vi "VCS Stop Recorder.vi"(8 "error in (no error)":errorcluster, 11 "axis in":cluster{"keyHandle":u32, "nodeId":u16}={"keyHandle"=0, "nodeId"=1}) -> (0 "error out":errorcluster, 3 "axis out":cluster{"keyHandle":u32, "nodeId":u16}={"keyHandle"=0, "nodeId"=1})   [LabVIEW 2017, in "maxonEPOS.lvlib"]
doc: "<B>VCS_StopRecorder</B> stops the data recording."
uses:
  Examples/maxonEPOS.lvlib
  Resources/EposCmd.dll
  SSI_Tool/InstrumentsInterfaces/Motordriver/maxon EPOS/Resources/EposCmd64.dll
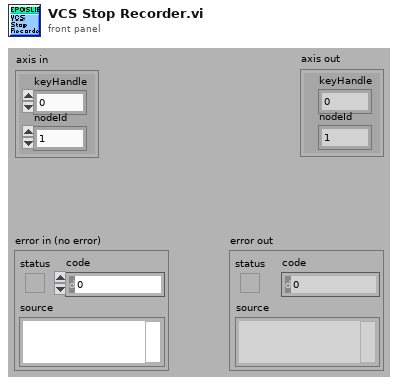
[diagram p1: front panel]
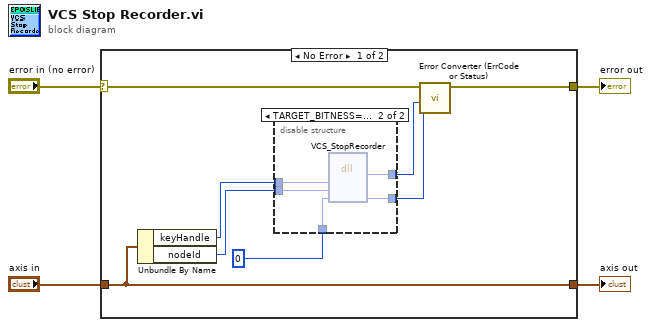
[diagram p0: block diagram]
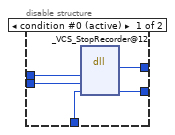
[diagram p2: hidden frame]
diagram:
  n1 = case shown="No Error" "error in (no error)" {
    selector: "error in (no error)" -> [w10 w23]
    tunnel: "axis in" -> [w12 w24]
    tunnel: [w12 w24] -> w3
    tunnel: [w11 w23] -> w2
    frame No Error {
      n2 = Unbundle By Name(w12) -> ("keyHandle"=w8:u32, "nodeId"=w9:u16)
      n3 = disable-structure shown="TARGET_BITNESS==64" {
        disable-tunnel: w9 -> [w17 w22]
        disable-tunnel: w8 -> [w16 w21]
        disable-tunnel: u32 0 ("pErrorCode") -> [w15 w20]
        disable-tunnel: [w14 w19] -> w6
        disable-tunnel: [w13 w18] -> w5
        frame condition #0 (active) {
          n4 = dll-call lib="C:/workspace/project/scancon/sw/SSI_Tool/InstrumentsInterfaces/Motordriver/maxon EPOS/Resources/EposCmd.dll" fn="_VCS_StopRecorder@12"("KeyHandle"=w16, "NodeId"=w17, "pErrorCode"=w15) -> ("Rückgabetyp"=w13:i32, "pErrorCode"=w14:u32)  [unwired: 5 in, 2 out]
        }
        frame condition #1 {
          n5 = dll-call lib="C:/Sources/LabView/maxon EPOS/Resources/EposCmd64.dll" fn="VCS_StopRecorder" ("EposCmd.dll:_VCS_StopRecorder@12")("KeyHandle"=w21, "NodeId"=w22, "pErrorCode"=w20) -> ("Rückgabetyp"=w18:i32, "pErrorCode"=w19:u32)  [unwired: 5 in, 2 out]
        }
      }
      n6 = call "Error Converter (ErrCode or Status).vi"("error code"=w6, "return type"=w5, "error in (no error)"=w10) -> ("error out"=w11:errorcluster)  [unwired: 7 in]
    }
    frame Error {
    }
  }
  "error out" <- w2
  "axis out" <- w3
